vi "MixAndDownsample_5782_10MhzPID.vi"(6 "sin0":fxp<+/-,16,0>, 9 "cos0":fxp<+/-,16,0>, 11 "signal 0":i16) -> (0 "data valid":bool, 1 "Q out":fxp<+/-,16,14>, 2 "I out":fxp<+/-,16,14>)   [LabVIEW 2013]
uses:
  <vilib>/rvi/FXPMathLib/FxpSub/XNode/nifxpmath_Sub.xnode
  <vilib>/rvi/FXPMathLib/sim/FxpSim.dll
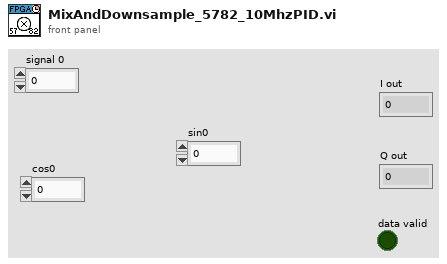
[diagram p1: front panel]
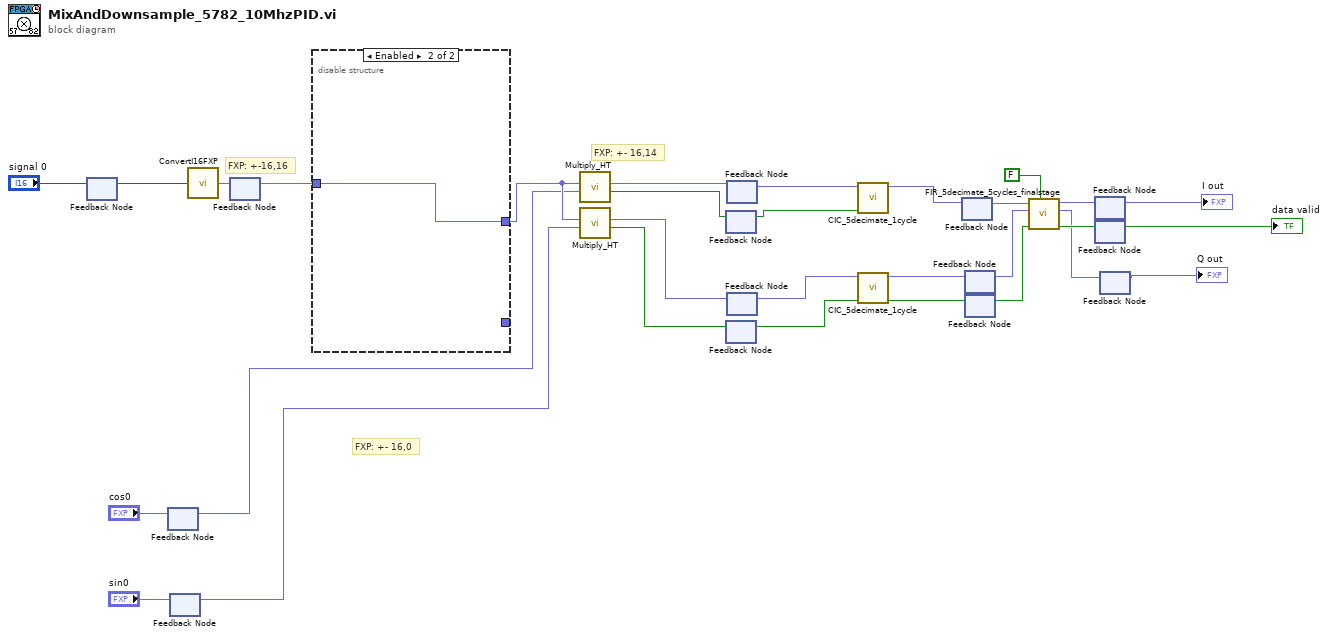
[diagram p0: block diagram]
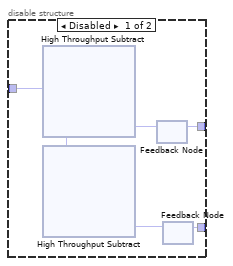
[diagram p2: hidden frame]
diagram:
  # "FXP: +- 16,14"
  # "FXP: +- 16,0"
  # "FXP: +-16,16"
  n1 = feedback #1() -> (w23:i16)  [unwired: 1 in]
  n2 = feedback-in #1("signal 0") -> ()
  n3 = feedback #2() -> (w20:fxp<+/-,16,0>)  [unwired: 1 in]
  n4 = feedback-in #2("cos0") -> ()
  n5 = feedback #3() -> (w19:fxp<+/-,16,0>)  [unwired: 1 in]
  n6 = feedback-in #3("sin0") -> ()
  n7 = call "ConvertI16FXP.vi"("I16"=w23) -> ("y"=w27:fxp<+/-,16,16>)
  n8 = feedback #4() -> (w26:fxp<+/-,16,16>)  [unwired: 1 in]
  n9 = feedback-in #4(w27) -> ()
  n10 = disable-structure shown="Enabled" {
    disable-tunnel: w26 -> [w37 w38]
    disable-tunnel: [w33 w38] -> w25
    disable-tunnel: [w31 _] -> _
    frame Disabled {
      n11 = xnode "High Throughput Subtract"("x"=w37) -> ("y"=w35:fxp<+/-,16,16>, "x-y"=w34:fxp<+/-,16,16>)
      n12 = xnode "High Throughput Subtract"("y"=w35) -> ("x"=w36:fxp<+/-,16,16>, "x-y"=w32:fxp<+/-,16,16>)
      n13 = feedback #5() -> (w33:fxp<+/-,16,16>)  [unwired: 1 in]
      n14 = feedback-in #5(w34) -> ()
      n15 = feedback #6() -> (w31:fxp<+/-,16,16>)  [unwired: 1 in]
      n16 = feedback-in #6(w32) -> ()
    }
    frame Enabled {
    }
  }
  n17 = call "Multiply_HT.vi"("DDS sample"=w20, "Signal sample"=w25) -> ("output valid"=w1:bool, "Output"=w18:fxp<+/-,16,14>)  [unwired: 8 in]
  n18 = call "Multiply_HT.vi"("DDS sample"=w19, "Signal sample"=w25) -> ("output valid"=w4:bool, "Output"=w17:fxp<+/-,16,14>)  [unwired: 8 in]
  n19 = feedback #7() -> (w2:bool)  [unwired: 1 in]
  n20 = feedback-in #7(w1) -> ()
  n21 = feedback #8() -> (w3:bool)  [unwired: 1 in]
  n22 = feedback-in #8(w4) -> ()
  n23 = feedback #9() -> (w9:fxp<+/-,16,14>)  [unwired: 1 in]
  n24 = feedback-in #9(w18) -> ()
  n25 = feedback #10() -> (w7:fxp<+/-,16,14>)  [unwired: 1 in]
  n26 = feedback-in #10(w17) -> ()
  n27 = call "CIC_5decimate_1cycle.vi"("valid in"=w2, "Data in"=w9) -> ("Data out"=w8:fxp<+/-,16,14>)  [unwired: 8 in, 1 out]
  n28 = call "CIC_5decimate_1cycle.vi"("valid in"=w3, "Data in"=w7) -> ("valid out"=w5:bool, "Data out"=w6:fxp<+/-,16,14>)  [unwired: 8 in]
  n29 = feedback #11() -> (w16:fxp<+/-,16,14>)  [unwired: 1 in]
  n30 = feedback-in #11(w8) -> ()
  n31 = feedback #12() -> (w15:fxp<+/-,16,14>)  [unwired: 1 in]
  n32 = feedback-in #12(w6) -> ()
  n33 = feedback #13() -> (w14:bool)  [unwired: 1 in]
  n34 = feedback-in #13(w5) -> ()
  n35 = call "FIR_5decimate_5cycles_finalstage.vi"("reset"=FALSE, "valid in"=w14, "Q in"=w15, "I in"=w16) -> ("valid out"=w29:bool, "Q out"=w12:fxp<+/-,16,14>, "I out"=w13:fxp<+/-,16,14>)  [unwired: 4 in, 1 out]
  n36 = feedback #14() -> (→"I out":fxp<+/-,16,14>)  [unwired: 1 in]
  n37 = feedback-in #14(w13) -> ()
  n38 = feedback #15() -> (→"data valid":bool)  [unwired: 1 in]
  n39 = feedback-in #15(w29) -> ()
  n40 = feedback #16() -> (→"Q out":fxp<+/-,16,14>)  [unwired: 1 in]
  n41 = feedback-in #16(w12) -> ()
